vi "Launch Hardware Settings Dialog.vi"(8 "error in (no error)":errorcluster, 9 "Device":string, 10 "Msmt":string, 11 "Controller in":refnum<class "Controller.lvclass">) -> (0 "error out":errorcluster, 3 "Controller out":refnum<class "Controller.lvclass">)   [LabVIEW 2017, in "Controller Actor.lvlib" / "Controller.lvclass"]
uses:
  Controller.lvclass
  C:/Program Files (x86)/National Instruments/LabVIEW 2017/vi.lib/ActorFramework/Actor/Actor.lvclass
  Hardware/HW Config/HW Configuration.lvclass/HW Configuration.ctl
  Controller.lvclass/Controller.ctl
  Hardware/HW Config/HW Configuration.lvclass
  Hardware/Hardware.lvclass
  <vilib>/ActorFramework/Actor/Actor.lvclass
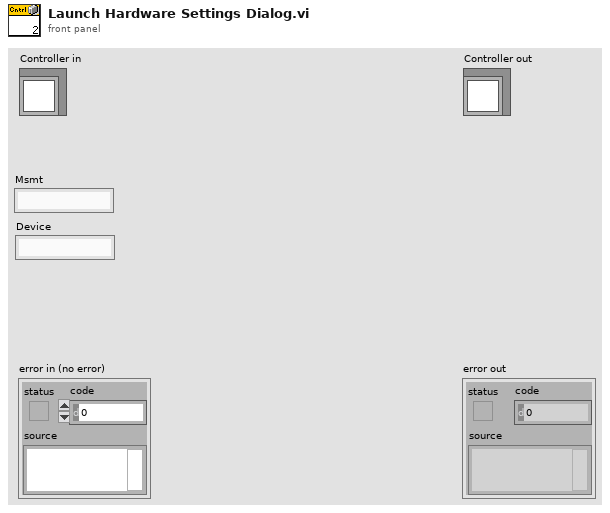
[diagram p1: front panel]
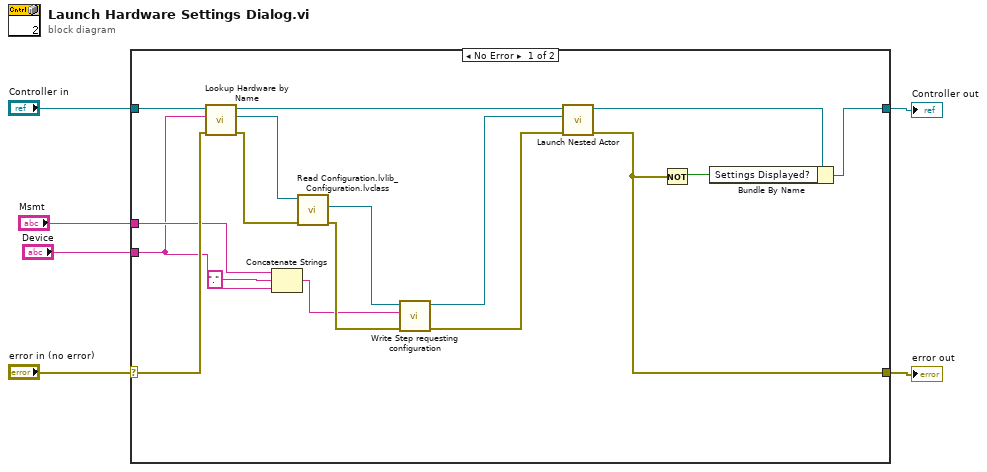
[diagram p0: block diagram]
diagram:
  n1 = case shown="No Error" "error in (no error)" {
    selector: "error in (no error)" -> [w19 w25]
    tunnel: [w12 w25] -> w5
    tunnel: [w22 w24] -> w3
    tunnel: "Controller in" -> [w20 w24]
    tunnel: "Device" -> [w10 _]
    tunnel: "Msmt" -> [w11 _]
    frame No Error {
      n2 = call "Lookup Hardware by Name.vi"("error in (no error)"=w19, "Device Name"=w10, "Controller in"=w20) -> ("error out"=w18:errorcluster, "Hardware.lvclass"=w21:refnum<class "Hardware.lvclass">, "Controller out"=w15:refnum<class "Controller.lvclass">)  [unwired: 6 in]
      n3 = Concatenate Strings(w11, "." ("string"), w10) -> (w8:string)
      n4 = call-dynamic "Read Configuration.lvlib_Configuration.lvclass.vi"("error in (no error)"=w18, "Hardware in"=w21) -> ("error out"=w16:errorcluster, "Hardware.lvlib:HW Configuration.lvclass"=w17:refnum<class "HW Configuration.lvclass">)  [unwired: 7 in, 1 out]
      n5 = call "Write Step requesting configuration.vi"("error in (no error)"=w16, "Step requesting configuration"=w8, "HW Configuration in"=w17) -> ("error out"=w13:errorcluster, "HW Configuration out"=w14:refnum<class "HW Configuration.lvclass">)  [unwired: 7 in]
      n6 = call <vilib>:"Launch Nested Actor.vi"("error in (no error)"=w13, "Nested Actor"=w14, "Caller Actor in"=w15) -> ("error out"=w12:errorcluster, "Caller Actor out"=w7:refnum<class "Controller.lvclass">)  [unwired: 6 in, 1 out]
      n7 = Not(x=w12) -> (.not. x?=w23:bool)
      n8 = Bundle By Name(cluster=w7, "Settings Displayed?"=w23) -> (w22:refnum<class "Controller.lvclass">)
    }
    frame Error {
    }
  }
  "error out" <- w5
  "Controller out" <- w3
